vi "test-SetGetControlValueSub.vi"() -> ()   [LabVIEW 2020]
panel:
  in  "Numeric":dbl
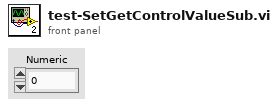
[diagram p1: front panel]
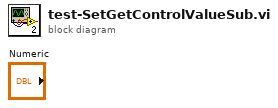
[diagram p0: block diagram]
diagram:
